vi "Forward Kinematics.vi"(8 "error in (no error)":errorcluster, 11 "Finger in":refnum<class "Finger.lvclass">) -> (0 "error out":errorcluster, 2 "T":T1=[[1.0, 0.0, 0.0, 0.0], [0.0, 1.0, 0.0, 0.0], [0.0, 0.0, 1.0, 0.0], [0.0, 0.0, 0.0, 1.0]], 3 "Finger out":refnum<class "Finger.lvclass">)   [LabVIEW 2013, in "Finger.lvclass"]
uses:
  Finger.lvclass
  <vilib>/Analysis/Matrix/Datatypes/RealMatrix.ctl
  Finger.lvclass/Finger.ctl
  <vilib>/Analysis/Matrix/Numeric/Multiply/Multiply - RM,RM.vi
  <vilib>/Analysis/Matrix/Numeric/Subtract/Subtract - RM,RM.vi
  <vilib>/Analysis/Matrix/Numeric/Add/Add - RM,RM.vi
  <vilib>/Analysis/Matrix/Numeric/Multiply/Multiply - RM,R.vi
  <vilib>/Analysis/Matrix/Numeric/Multiply/Multiply - R,RM.vi
  <vilib>/Analysis/Matrix/Numeric/Conversions/Array To Matrix - RA.vi
  <vilib>/Analysis/Matrix/Numeric/Conversions/Array To Matrix - RA2.vi
  <vilib>/Analysis/Matrix/NI_Matrix.lvlib
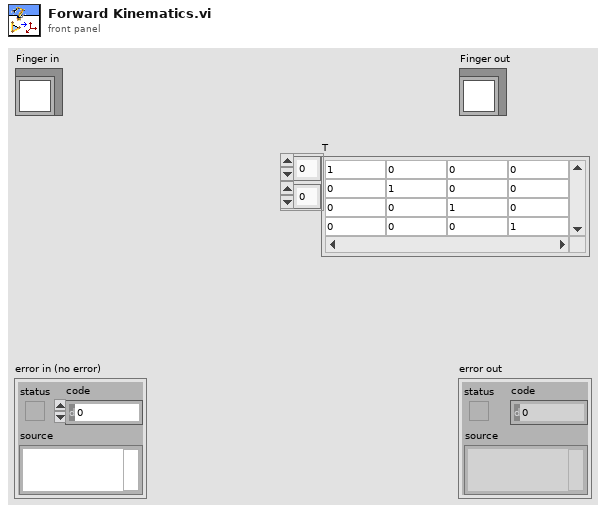
[diagram p1: front panel]
types:
  T1 = typedef "NI_Matrix.lvlib/RealMatrix.ctl" = dbl[][]
  T2 = typedef "NI_Robotics_Link.lvclass/Joint Type.ctl" = enum16{"Revolute", "Prismatic"}
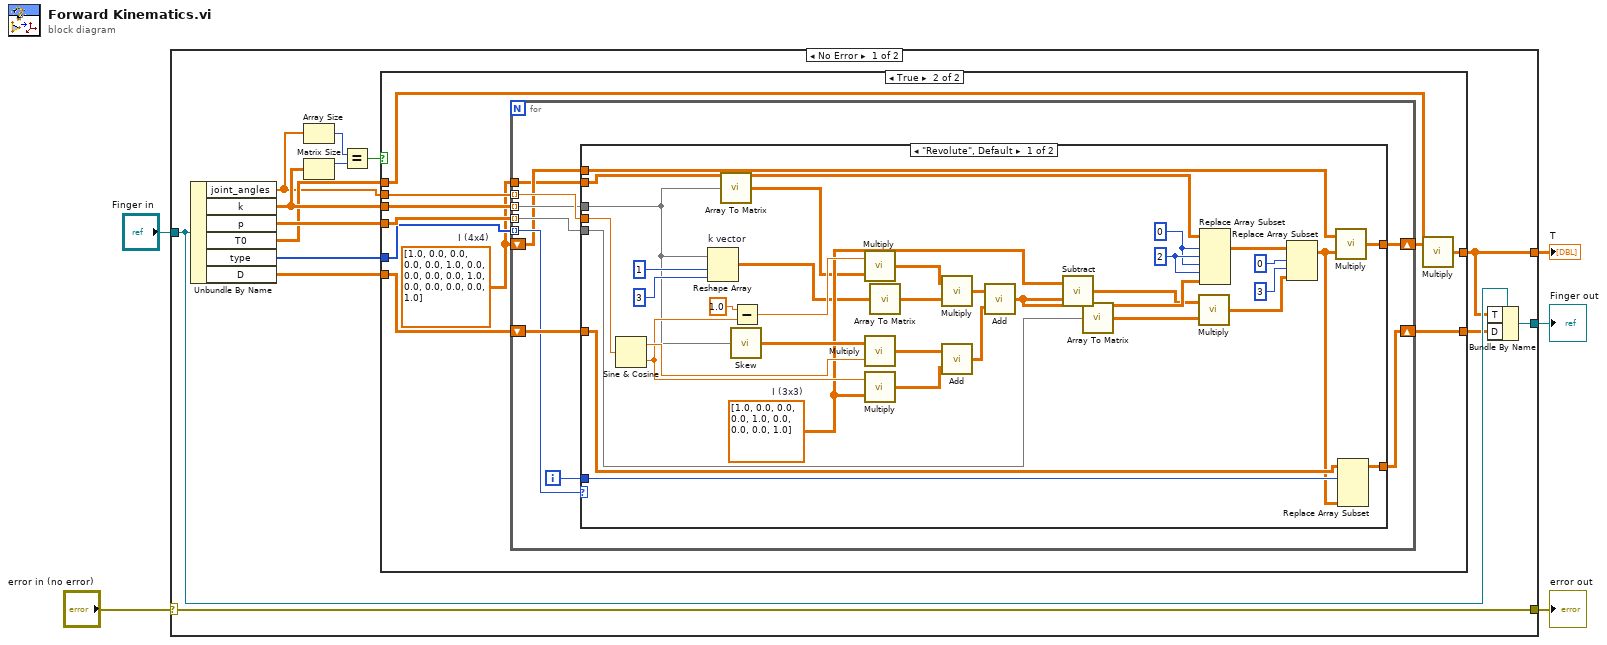
[diagram p0: block diagram]
diagram:
  n1 = case shown="No Error" "error in (no error)" {
    selector: "error in (no error)" -> [w19 w76]
    tunnel: [w19 w76] -> w4
    tunnel: [w9 w75] -> w2
    tunnel: "Finger in" -> [w11 w75]
    tunnel: [w10 _] -> w1
    frame No Error {
      n2 = Unbundle By Name(w11) -> ("joint_angles"=w12:dbl[], "k"=w18:T1, "p"=w17:T1, "T0"=w16:T1, "type"=w6:T2[], "D"=w7:dbl[][][])
      n3 = Array Size(array=w12) -> (size(s)=w15:i32)
      n4 = Matrix Size(0:w18) -> (1:w14:i32)  [unwired: 1 out]
      n5 = Equal?(x=w15, y=w14) -> (x = y?=w13:bool)
      n6 = case shown="True" w13 {
        tunnel: w12 -> [_ w29]
        tunnel: w17 -> [_ w28]
        tunnel: w18 -> [_ w27]
        tunnel: [_ w25] -> w10
        tunnel: w16 -> [_ w24]
        tunnel: w7 -> [_ w23]
        tunnel: [_ w22] -> w8
        tunnel: w6 -> [_ w21]
        frame False {
        }
        frame True {
          w20 = T1 [[1.0, 0.0, 0.0, 0.0], [0.0, 1.0, 0.0, 0.0], [0.0, 0.0, 1.0, 0.0], [0.0, 0.0, 0.0, 1.0]]  # I (4x4)
          n7 = for {
            tunnel: w29 -> [w39] mode=indexing
            tunnel: w28 -> [w36] mode=indexing
            tunnel: w27 -> [w37] mode=indexing
            shift-right: [w38] -> w26
            shift-left: w20 -> [w31]
            shift-right: [w33] -> w22
            shift-left: w23 -> [w35]
            tunnel: w21 -> [w32] mode=indexing
            tunnel: w20 -> [w30]
            i -> [w34]
            n8 = case shown="\"Revolute\", Default" w32 {
              tunnel: w39 -> [w74 _]
              tunnel: [w58 _] -> w38
              tunnel: w37 -> [w54 _]
              tunnel: w36 -> [w51 _]
              tunnel: w35 -> [w45 _]
              tunnel: w34 -> [w44 _]
              tunnel: [w43 _] -> w33
              tunnel: w30 -> [w41 _]
              tunnel: w31 -> [w40 _]
              frame "Revolute", Default {
                w63 = 2 ("row N")
                w62 = 0 ("row 1")
                w61 = T1 [[1.0, 0.0, 0.0], [0.0, 1.0, 0.0], [0.0, 0.0, 1.0]]  # I (3x3)
                n9 = Sine & Cosine(0:w74) -> (1:w72:dbl, 2:w68:dbl)
                n10 = Reshape Array "k vector"(w54, 1 ("dimension size"), 3 ("dimension size")) -> (w52:dbl[][])
                n11 = call-poly <vilib>:"Array To Matrix.vi"("Real 1D Array"=w54) -> ("Real Matrix (Column Vector)"=w57:T1)
                n12 = call "Skew.vi"("k"=w54) -> ("M"=w73:T1)
                n13 = Subtract(x=1.0, y=w68) -> (x-y=w67:dbl)
                n14 = call-poly <vilib>:"Multiply.vi"("Real Matrix A"=w57, "Real Scalar c"=w67) -> ("c * A"=w66:T1)
                n15 = call-poly <vilib>:"Multiply.vi"("Real Scalar c"=w72, "Real Matrix A"=w73) -> ("A * c"=w70:T1)
                n16 = call-poly <vilib>:"Multiply.vi"("Real Matrix A"=w61, "Real Scalar c"=w68) -> ("c * A"=w71:T1)
                n17 = call-poly <vilib>:"Array To Matrix.vi"("Real 2D Array"=w52) -> ("Real Matrix"=w53:T1)
                n18 = call-poly <vilib>:"Multiply.vi"("Real Matrix B"=w53, "Real Matrix A"=w66) -> ("A * B"=w64:T1)
                n19 = call-poly <vilib>:"Add.vi"("Real Matrix B"=w71, "Real Matrix A"=w70) -> ("A + B"=w65:T1)
                n20 = call-poly <vilib>:"Add.vi"("Real Matrix B"=w65, "Real Matrix A"=w64) -> ("A + B"=w60:T1)
                n21 = call-poly <vilib>:"Subtract.vi"("Real Matrix B"=w60, "Real Matrix A"=w61) -> ("A - B"=w59:T1)
                n22 = call-poly <vilib>:"Array To Matrix.vi"("Real 1D Array"=w51) -> ("Real Matrix (Column Vector)"=w50:T1)
                n23 = call-poly <vilib>:"Multiply.vi"("Real Matrix B"=w50, "Real Matrix A"=w59) -> ("A * B"=w48:T1)
                n24 = Replace Array Subset(array=w41, new element=w60, index (dim 0)=w62, index (dim 1)=w63, index (dim 2)=w62, index (dim 3)=w63) -> (w49:T1)
                n25 = Replace Array Subset(array=w49, new element=w48, index (row)=0 ("disabled index (row)"), index (col)=3 ("disabled index (col)")) -> (w42:T1)
                n26 = call-poly <vilib>:"Multiply.vi"("Real Matrix B"=w42, "Real Matrix A"=w40) -> ("A * B"=w58:T1)
                n27 = Replace Array Subset(array=w45, new element=w42, index (dim 0)=w44) -> (w43:dbl[][][])  [unwired: 2 in]
              }
              frame "Prismatic" {
                # "TODO: Implement calculation of D for prismatic joints"
              }
            }
          }
          n28 = call-poly <vilib>:"Multiply.vi"("Real Matrix B"=w24, "Real Matrix A"=w26) -> ("A * B"=w25:T1)
        }
      }
      n29 = Bundle By Name(cluster=w11, "T"=w10, "D"=w8) -> (w9:refnum<class "Finger.lvclass">)
    }
    frame Error {
    }
  }
  "error out" <- w4
  "Finger out" <- w2
  "T" <- w1
